vi "Extract TDMS FGEN Info.vi"(8 "error in (no error)":errorcluster, 10 "TDMS Name Mapping":T2, 11 "TDMS File Path":string) -> (0 "error out":errorcluster, 3 "TDMS FGEN Info":T1)   [LabVIEW 2025, in "FGEN Arb Sequence Mode.lvclass"]
uses:
  FGEN Arb Sequence Mode.lvclass
  52e7fa97-1c4b-4cb3-8030-13428e347abd.vi
  52e7fa97-1c4b-4cb3-8030-13428e347abd.vi/d4db2432-cc9c-482c-8957-dac855435ef6.vi
  52e7fa97-1c4b-4cb3-8030-13428e347abd.vi/86fbf154-bd7b-49a2-8ab2-a837b2a95f24.vi
  52e7fa97-1c4b-4cb3-8030-13428e347abd.vi/3b95b01e-1ec2-4565-bcd9-7606a5281010.vi
  52e7fa97-1c4b-4cb3-8030-13428e347abd.vi/96a08935-737a-44b2-979c-a81d56408f7e.vi
  52e7fa97-1c4b-4cb3-8030-13428e347abd.vi/d4db2432-cc9c-482c-8957-dac855435ef6.vi/6eaecd13-6e48-4772-a921-b51ebdf84d88.vi
  52e7fa97-1c4b-4cb3-8030-13428e347abd.vi/d4db2432-cc9c-482c-8957-dac855435ef6.vi/d2d5f2b7-06f4-47f6-971c-049c3fdbb653.vi
  52e7fa97-1c4b-4cb3-8030-13428e347abd.vi/3b95b01e-1ec2-4565-bcd9-7606a5281010.vi/6eaecd13-6e48-4772-a921-b51ebdf84d88.vi
  52e7fa97-1c4b-4cb3-8030-13428e347abd.vi/3b95b01e-1ec2-4565-bcd9-7606a5281010.vi/d2d5f2b7-06f4-47f6-971c-049c3fdbb653.vi
  52e7fa97-1c4b-4cb3-8030-13428e347abd.vi/96a08935-737a-44b2-979c-a81d56408f7e.vi/6eaecd13-6e48-4772-a921-b51ebdf84d88.vi
  52e7fa97-1c4b-4cb3-8030-13428e347abd.vi/96a08935-737a-44b2-979c-a81d56408f7e.vi/d2d5f2b7-06f4-47f6-971c-049c3fdbb653.vi
  <vilib>/Utility/error.llb/Error Cluster From Error Code.vi
  <vilib>/Comparison/Less/Less Functor/Less Functor.lvclass
  <vilib>/ErrorRing/Error Ring.xnode
  FGEN Arb Sequence Mode.lvclass/FGEN Arb Sequence Mode.ctl
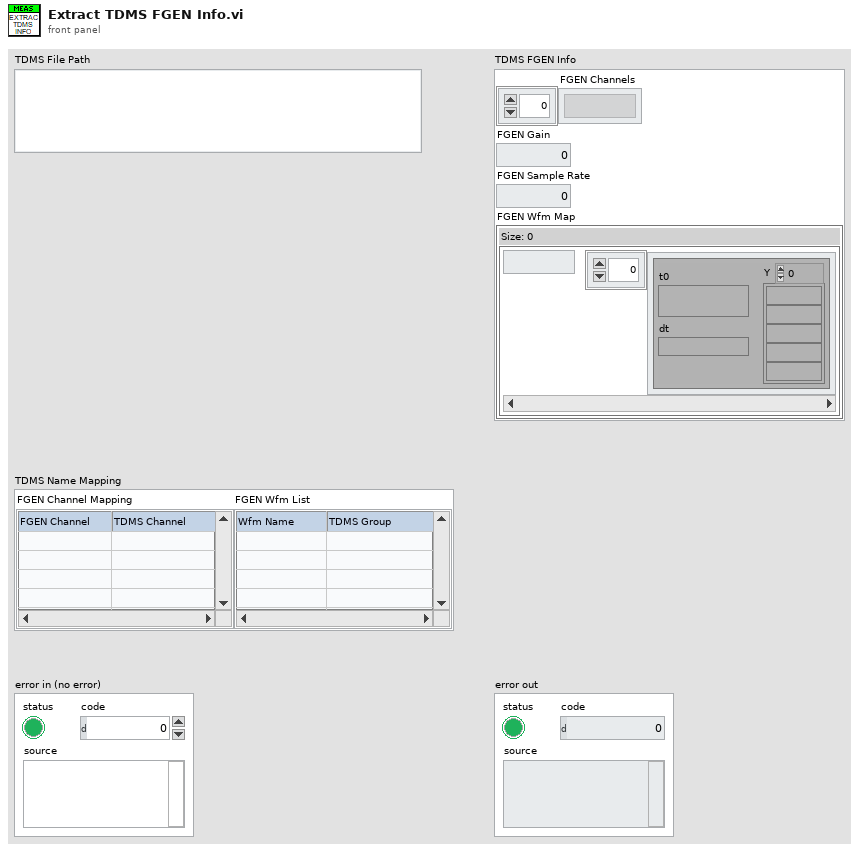
[diagram p1: front panel]
types:
  T1 = cluster{"FGEN Channels":string[], "FGEN Gain":dbl, "FGEN Sample Rate":dbl, "FGEN Wfm Map":map{string, waveform(dbl)[]}}
  T2 = cluster{"FGEN Channel Mapping":string[][], "FGEN Wfm List":string[][]}
  T3 = enum16{"open", "open or create", "create or replace", "create", "open (read-only)"}
  T4 = enum16{"Error or Wfm Not Found", "Not all Chns Found", "All Found"}
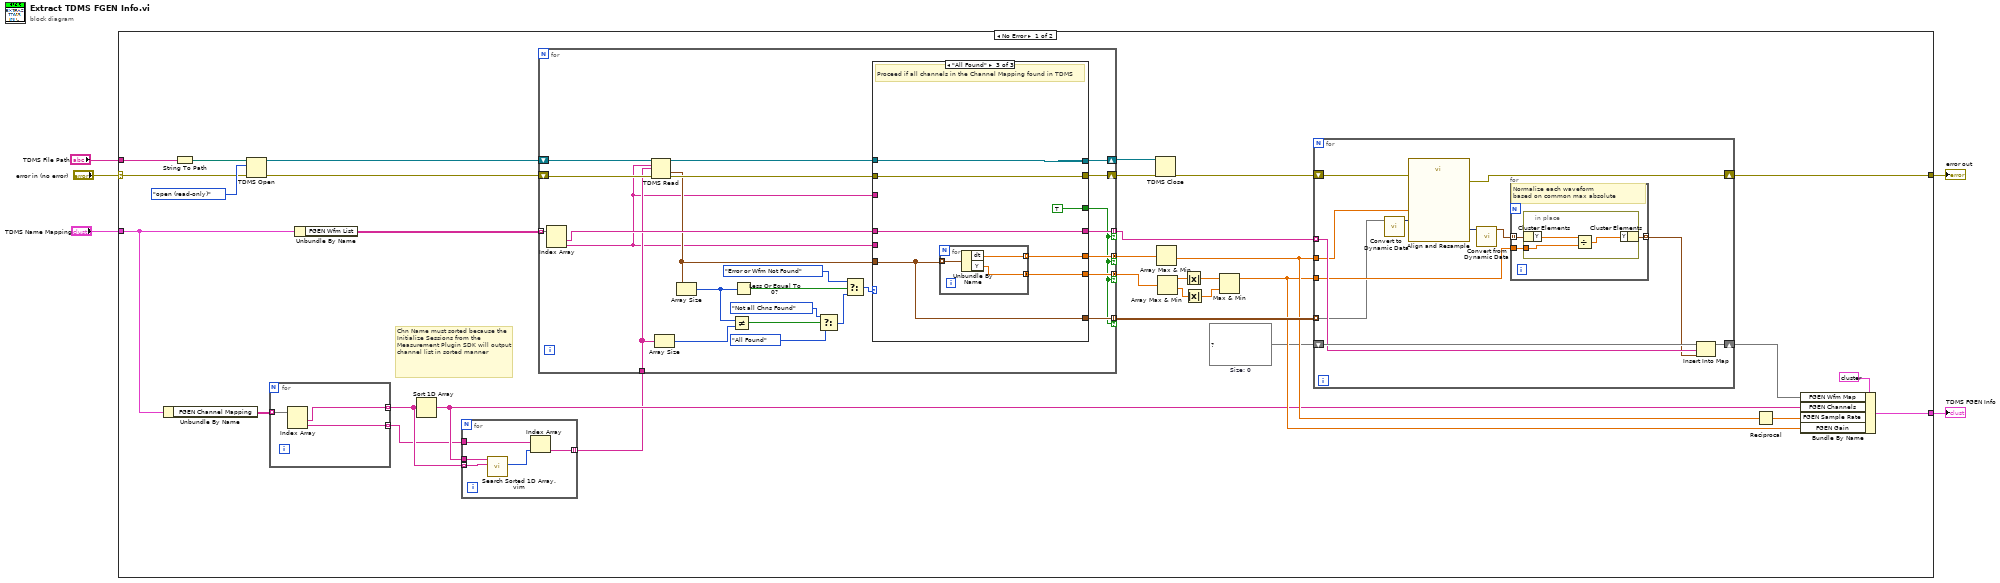
[diagram p0: block diagram]
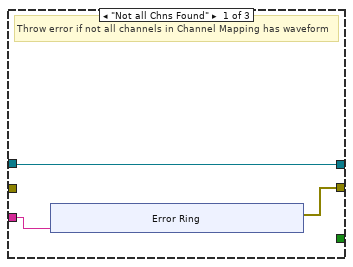
[diagram p2: hidden frame]
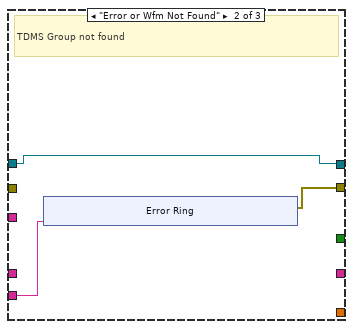
[diagram p3: hidden frame]
diagram:
  n1 = case shown="No Error" "error in (no error)" {
    selector: "error in (no error)" -> [w29 w119]
    tunnel: "TDMS File Path" -> [w35 _]
    tunnel: [w24 w119] -> w4
    tunnel: "TDMS Name Mapping" -> [w7 _]
    tunnel: [w18 _] -> w1
    frame No Error {
      w9 = map{string, waveform(dbl)[]} {}  # Size: 0
      # "Chn Name must sorted because the Initialize Sessions from the Measurement Plugin SDK will output channel list in sorted manner"
      n2 = Unbundle By Name(w7) -> ("FGEN Channel Mapping"=w36:string[][])
      n3 = String To Path(string=w35) -> (path=w23:path)
      n4 = TDMS Open(8:w29, 10:T3."open (read-only)" ("operation (0:open)"), 11:w23) -> (0:w33:errorcluster, 3:w34:refnum<k34>)  [unwired: 4 in]
      n5 = for {
        tunnel: w36 -> [w118] mode=indexing
        tunnel: [w117] -> w12 mode=indexing
        tunnel: [w116] -> w11 mode=indexing
        n6 = Index Array(array=w118) -> (element #1=w117:string, element #2=w116:string)  [unwired: 2 in]
      }
      n7 = Unbundle By Name(w7) -> ("FGEN Wfm List"=w37:string[][])
      n8 = Sort 1D Array(array=w12) -> (sorted array=w13:string[])
      n9 = for {
        tunnel: w13 -> [w115]
        tunnel: w12 -> [w114] mode=indexing
        tunnel: w11 -> [w113]
        tunnel: [w111] -> w10 mode=indexing
        n10 = call "Search Sorted 1D Array.vim"("element"=w114, "sorted 1D array"=w115) -> ("nearest index"=w112:i32)  [unwired: 8 in, 1 out]
        n11 = Index Array(array=w113, index=w112) -> (element=w111:string)
      }
      n12 = for {
        tunnel: w37 -> [w80] mode=indexing
        tunnel: [w72] -> w25 mode=indexing if=w59
        shift-right: [w61] -> w30
        shift-left: w33 -> [w78]
        shift-right: [w76] -> w31
        shift-left: w34 -> [w79]
        tunnel: [w75] -> w27 mode=indexing if=w59
        tunnel: [w74] -> w28 mode=concatenating if=w59
        tunnel: [w60] -> w16 mode=concatenating if=w59
        tunnel: w10 -> [w57]
        n13 = Index Array(array=w80) -> (element #1=w73:string, element #2=w56:string)  [unwired: 2 in]
        n14 = TDMS Read(0:w79, 5:w56, 7:w57, 11:w78) -> (4:w77:refnum<k34>, 10:w70:waveform(dbl)[], 15:w71:errorcluster)  [unwired: 4 in, 3 out]
        n15 = Array Size(array=w57) -> (size(s)=w58:i32)
        n16 = Array Size(array=w70) -> (size(s)=w67:i32)
        n17 = Not Equal?(x=w67, y=w58) -> (x != y?=w64:bool)
        n18 = Less Or Equal To 0?(x=w67) -> (x <= 0?=w68:bool)
        n19 = Select(t=T4."Not all Chns Found", s=w64, f=T4."All Found") -> (s? t:f=w65:T4)
        n20 = Select(t=T4."Error or Wfm Not Found", s=w68, f=w65) -> (s? t:f=w62:T4)
        n21 = case shown="\"All Found\"" w62 {
          tunnel: w71 -> [_ _ w104]
          tunnel: w77 -> [w83 w93 w107]
          tunnel: [w83 w93 w107] -> w76
          tunnel: w56 -> [w82 _ _]
          tunnel: [_ _ w101] -> w75
          tunnel: [_ _ w106] -> w74
          tunnel: w70 -> [_ _ w101]
          tunnel: w73 -> [_ _ w105]
          tunnel: [_ _ w105] -> w72
          tunnel: [_ _ TRUE] -> w59
          tunnel: [w81 w92 w104] -> w61
          tunnel: [_ _ w102] -> w60
          tunnel: w56 -> [_ w91 _]
          frame "Not all Chns Found" {
            # "Throw error if not all channels in Channel Mapping has waveform"
            n22 = xnode "Error Ring"("parameter 0"=w82) -> ("error out"=w81:errorcluster)
          }
          frame "Error or Wfm Not Found" {
            # "TDMS Group not found"
            n23 = xnode "Error Ring"("parameter 0"=w91) -> ("error out"=w92:errorcluster)
          }
          frame "All Found" {
            # "Proceed if all channels in the Channel Mapping found in TDMS"
            n24 = for {
              tunnel: w101 -> [w110] mode=indexing
              tunnel: [w109] -> w106 mode=indexing
              tunnel: [w108] -> w102 mode=concatenating
              n25 = Unbundle By Name(w110) -> ("dt"=w109:dbl, "Y"=w108:dbl[])
            }
          }
        }
      }
      n26 = TDMS Close(8:w30, 11:w31) -> (0:w26:errorcluster)  [unwired: 1 out]
      n27 = Array Max & Min(array=w28) -> (min value=w15:dbl)  [unwired: 3 out]
      n28 = Array Max & Min(array=w16) -> (max value=w20:dbl, min value=w19:dbl)  [unwired: 2 out]
      n29 = Absolute Value(x=w20) -> (abs(x)=w22:dbl)
      n30 = Absolute Value(x=w19) -> (abs(x)=w21:dbl)
      n31 = Max & Min(x=w22, y=w21) -> (max(x,y)=w14:dbl)  [unwired: 1 out]
      n32 = for {
        tunnel: w27 -> [w39] mode=indexing
        shift-right: [w38] -> w8
        shift-left: w9 -> [w49]
        tunnel: w15 -> [w43]
        shift-right: [w47] -> w24
        shift-left: w26 -> [w48]
        tunnel: w25 -> [w44] mode=indexing
        tunnel: w14 -> [w40]
        n33 = call "Convert to Dynamic Data"("Array of Waveforms"=w39) -> ("Dynamic Data Type"=w46:dynamicdata)  [unwired: 3 in]
        n34 = call "Align and Resample"("dt"=w43, "error in (no error)"=w48, "Signals"=w46) -> ("error out"=w47:errorcluster, "Resampled Signals"=w45:dynamicdata)  [unwired: 6 in, 1 out]
        n35 = call "Convert from Dynamic Data"("Dynamic Data Type"=w45) -> ("Array of Waveform"=w42:waveform(dbl)[])  [unwired: 3 in]
        n36 = for {
          tunnel: w42 -> [w52] mode=indexing
          tunnel: [w51] -> w41 mode=indexing
          tunnel: w40 -> [w50]
          # "Normalize each waveform\nbased on common max absolute"
          n37 = in-place {
            in-place-border: w50 -> [w53]
            n38 = in-place-cluster #1(w52) -> ("Y"=w55:dbl[])
            n39 = Divide(x=w55, y=w53) -> (x/y=w54:dbl[])
            n40 = in-place-cluster #1("Y"=w54) -> (w51:waveform(dbl))
          }
        }
        n41 = Insert Into Map(map in=w49, key=w44, value=w41) -> (map out=w38:map{string, waveform(dbl)[]})  [unwired: 2 out]
      }
      n42 = Reciprocal(x=w15) -> (1/x=w17:dbl)
      n43 = Bundle By Name(cluster=T1 {"FGEN Channels"=[], "FGEN Gain"=0.0, "FGEN Sample Rate"=0.0, "FGEN Wfm Map"={}} ("TDMS FGEN Info"), "FGEN Wfm Map"=w8, "FGEN Channels"=w13, "FGEN Sample Rate"=w17, "FGEN Gain"=w14) -> (w18:T1)
    }
    frame Error {
    }
  }
  "error out" <- w4
  "TDMS FGEN Info" <- w1
